vi "Update Scan Distance.vi"(9 "scan angle":dbl, 10 "new scan distance":dbl, 11 "scan angles in":T1) -> (3 "scan angles out":T1)   [LabVIEW 2017, in "NI_Robotics_Scan Angles.lvlib"]
uses:
  <vilib>/robotics/Utilities/Scan Angles/NI_Robotics_Scan Angles.lvlib
  <vilib>/robotics/Utilities/Scan Angles/Scan Angle Data.ctl
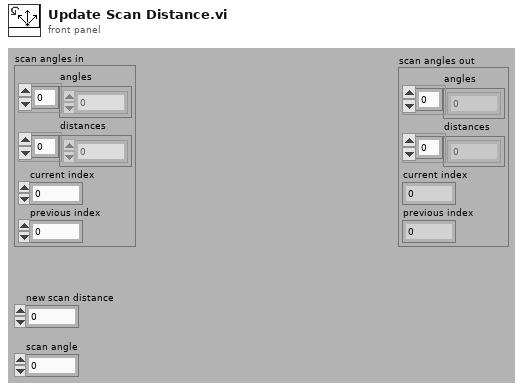
[diagram p1: front panel]
types:
  T1 = typedef "NI_Robotics_Scan Angles.lvlib/Scan Angle Data.ctl" = cluster{"angles":dbl[], "distances":dbl[], "current index":i32, "previous index":i32}
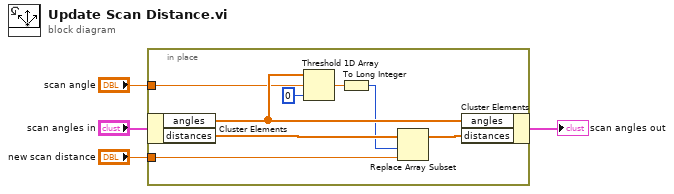
[diagram p0: block diagram]
diagram:
  n1 = in-place {
    in-place-border: "scan angle" -> [w6]
    in-place-border: "new scan distance" -> [w5]
    n2 = in-place-cluster #1("scan angles in") -> ("angles"=w11:dbl[], "distances"=w9:dbl[])
    n3 = Threshold 1D Array(1:0 ("start index (0)"), 2:w6, 3:w11) -> (0:w10:dbl)
    n4 = To Long Integer(number=w10) -> (32bit integer=w7:i32)
    n5 = Replace Array Subset(array=w9, new element=w5, index=w7) -> (w8:dbl[])
    n6 = in-place-cluster #1("angles"=w11, "distances"=w8) -> (→"scan angles out":T1)
  }
